vi "InitialiseProbeplan.vi"(8 "error in (no error)":errorcluster, 11 "ProbeStationControl in":refnum<class "ProbeStationControl.lvclass">) -> (0 "error out":errorcluster, 3 "ProbeStationControl out":refnum<class "ProbeStationControl.lvclass">)   [LabVIEW 2019]
doc: "General utility to initialise, generate, test and execute probe plans."
uses:
  InstrControl/ProbeStationControl/ProbeStationControl.lvclass
  ProbePlanParams.vi
  general_VIs/globals/QC_MeasurementSetup.vi
panel:
  in  "Continue":bool
  in  "New Sensor":bool
  in  "Single Needle":bool
  in  "Probe Card Channels":i32=32
  in  "Strip No.":u16(ring)
  out "Probeplan:":string
  in  "Region":u16(ring)
  in  "Chuck":bool caption="Chuck\nDOWN"
  in  "New Button":bool
  in  "Jump Button":bool
  out "Chuck Up/Down check":bool
  # "Probeplan"
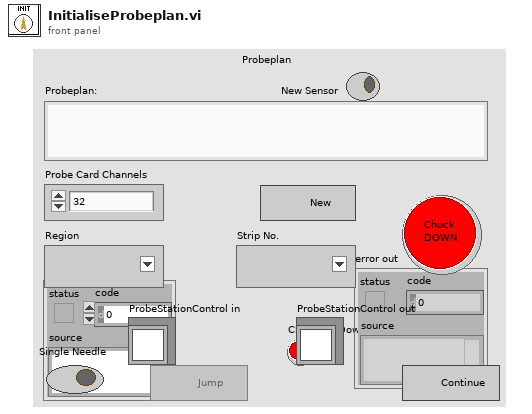
[diagram p1: front panel]
types:
  T1 = cluster{"Strip Number OUT":i32, "X0":i32, "Y0":i32, "X1":i32, "Y1":i32, "Xref":dbl, "Yref":dbl, "ProbePlan type":u32, "Inner pads offset":ext, "Outer pads offset":ext, "l_inner":ext, "l_outer":ext, "strip numbering":u16, "Device Orientation":ext, "Stagger offset":i32, "Yoffset":dbl, "Strip pitch":dbl, "Fiducail separation":dbl, "Radius":ext, "Relative strip angles":dbl, "Probeplan description":string, "ProbePlan array":cluster{"Region":string, "ProbePoints":cluster{"X":dbl, "Y":dbl, "Label":string, "CardViable?":bool}[]}[], "Test ProbePoints":cluster{"Regions Enabled":bool[], "From index":u32[], "To index":u32[]}}
  T2 = cluster{"Bias Supply":refnum<class "SupplyControl.lvclass">, "SMU":refnum<class "SupplyControl.lvclass">, "LCR":refnum<class "LCRControl.lvclass">, "Probe Card Channels":i32, "Bias Voltage [V]":dbl, "First strip":i32, "Last strip":i32, "Base Voltage [V]":dbl, "Base Ramp Step [V]":dbl, "Base Ramp Interval [ms]":u32, "High Voltage [V]":dbl, "High Ramp Step [V]":dbl, "High Ramp Interval [ms]":u32, "AC frequency [Hz]":i32, "AC amplitude [V]":dbl, "RC Configuration":u16, "Single Needle":bool, "Temperature Readout":enum16{"Read Arduino", "Enter manually"}, "Arduino":refnum<class "ArduinoControl.lvclass">, "Fraction of good strips [%]":dbl, "ProbeStation":refnum<class "ProbeStationControl.lvclass">, "Switching":refnum<class "Switching.lvclass">, "Matrix used?":bool, "Matrix X Channels":cluster{"Bias Supply / SMU LO":i32, "Bias Supply / SMU HI":i32, "CV Box LO":i32, "CV Box HI":i32, "CV Box LO IN":i32, "CV Box HI IN":i32, "Volt meter LO":i32, "Volt meter HI":i32, "Mux1 C1":i32, "Mux1 C2":i32, "Mux2 C1":i32, "Mux2 C2":i32}, "Pinholes Y/N":bool, "Capacitance Y/N":bool, "Resistance Y/N":bool, "Bias Supply Name":string, "SMU Name":string, "LCR Name":string}
  T3 = cluster{"Region":string, "ProbePoints":cluster{"X":dbl, "Y":dbl, "Label":string, "CardViable?":bool}[]}[]
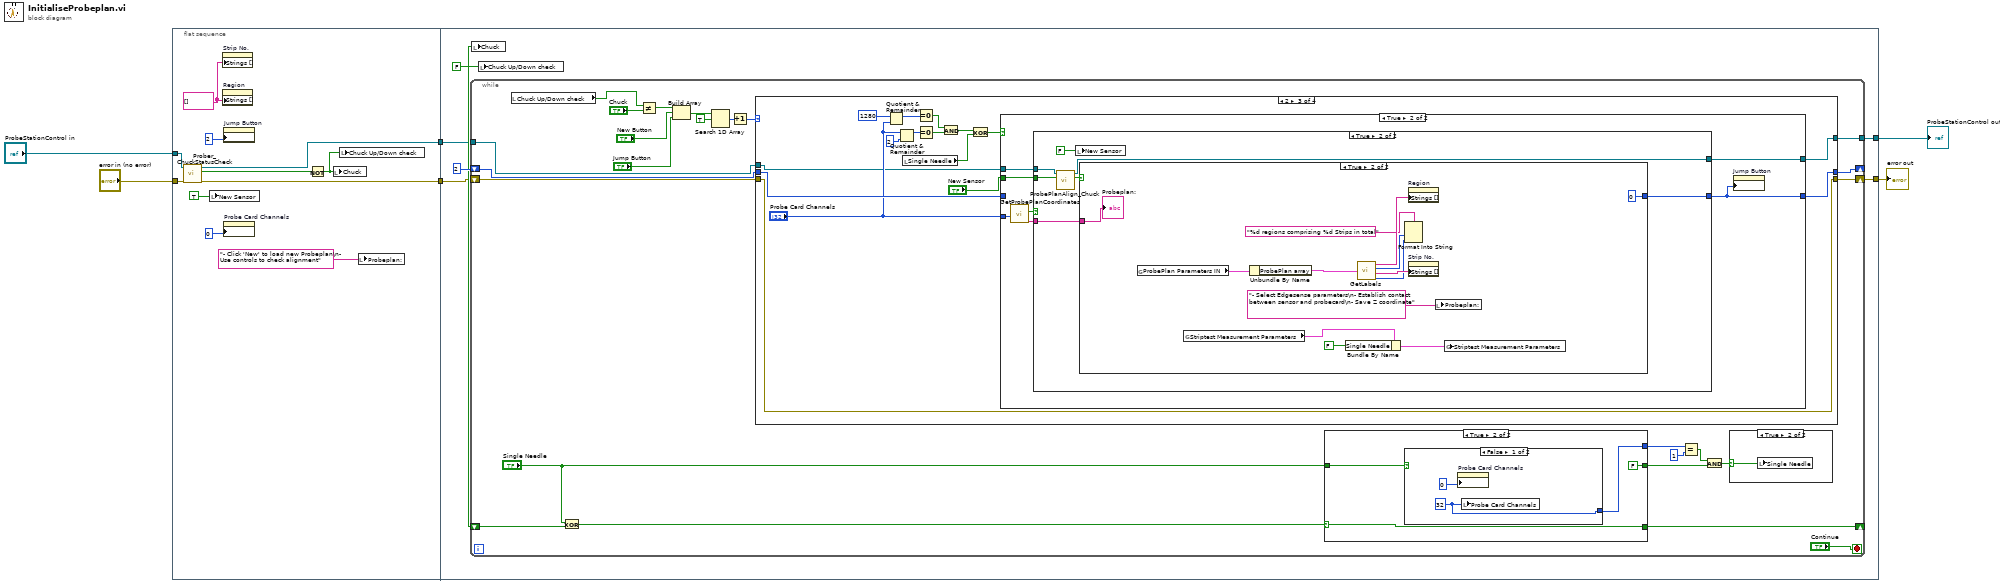
[diagram p0: block diagram]
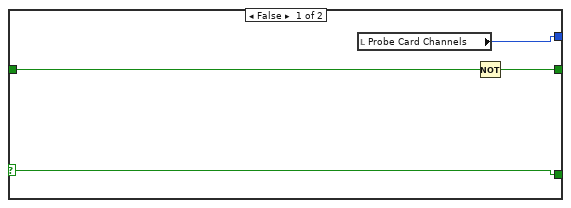
[diagram p3: hidden frame]
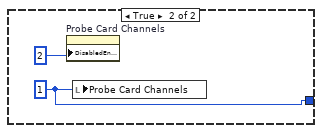
[diagram p4: hidden frame]
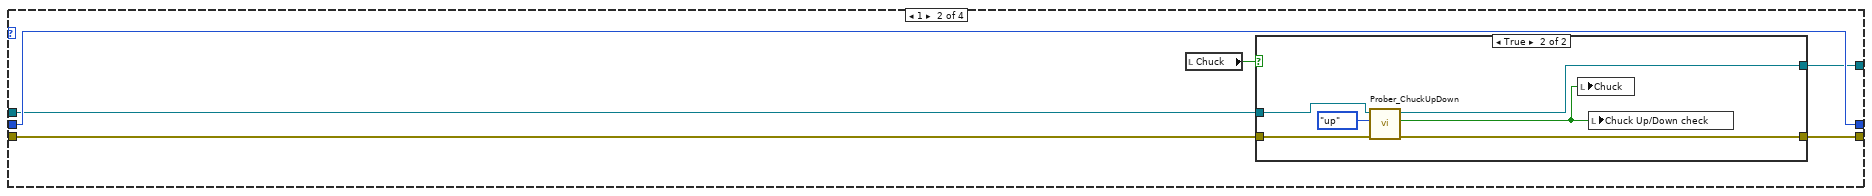
[diagram p6: hidden frame]
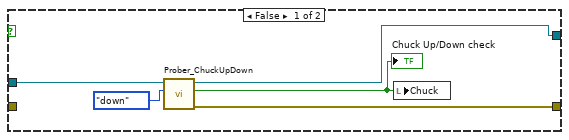
[diagram p7: hidden frame]
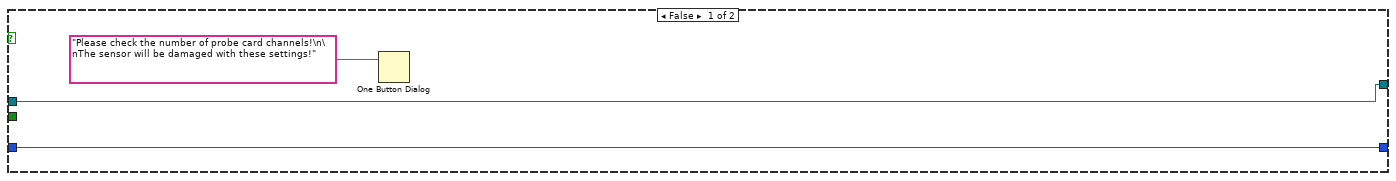
[diagram p8: hidden frame]
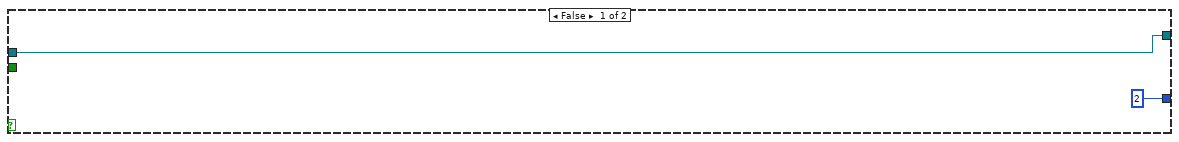
[diagram p9: hidden frame]
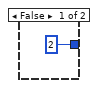
[diagram p10: hidden frame]
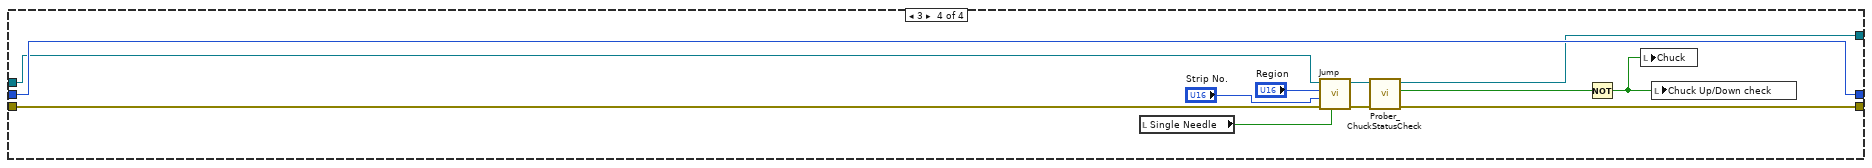
[diagram p11: hidden frame]
diagram:
  n1 = flat-sequence {
    tunnel: "ProbeStationControl in" -> [w11]
    tunnel: [w7] -> w3
    tunnel: "error in (no error)" -> [w9]
    tunnel: [w8] -> w2
    tunnel: w3 -> [w21]
    tunnel: [w20] -> w5
    tunnel: w2 -> [w19]
    tunnel: [w18] -> w1
    frame #0 {
      w15 = string[] []
      n2 = call-dynamic "Prober_ChuckStatusCheck.vi"("error in (no error)"=w9, "ProbeStationControl in"=w11) -> ("error out"=w8:errorcluster, "Chuck at CONTACT?"=w13:bool, "ProbeStationControl out"=w7:refnum<class "ProbeStationControl.lvclass">)  [unwired: 7 in]
      n3 = local write "New Sensor"(TRUE) -> ()
      n4 = property on="Strip No." class="Ring (strict)"("Strings []"=w15) -> ()  [unwired: 2 in, 2 out]
      n5 = property on="Region" class="Ring (strict)"("Strings []"=w15) -> ()  [unwired: 2 in, 2 out]
      n6 = property on="Jump Button" class="Bool"("DisabledEnum"=2) -> ()  [unwired: 2 in, 2 out]
      n7 = property on="Probe Card Channels" class="DigNum (strict)"("DisabledEnum"=0) -> ()  [unwired: 2 in, 2 out]
      n8 = Not(x=w13) -> (.not. x?=w12:bool)
      n9 = local write "Chuck"(w12) -> ()
      n10 = local write "Chuck Up/Down check"(w12) -> ()
      n11 = local write "Probeplan:"("- Click 'New' to load new Probeplan\n- Use controls to check alignment") -> ()
    }
    frame #1 {
      w22 = FALSE
      n12 = while {
        shift-right: [w41] -> _
        shift-left: 2 -> [w42]
        shift-right: [w29] -> _
        shift-left: w22 -> [w30]
        tunnel: w21 -> [w27]
        tunnel: [w26] -> w20
        shift-right: [w24] -> w18
        shift-left: w19 -> [w25]
        stop <- "Continue" stop-if-true
        n13 = local read "Chuck Up/Down check"() -> (w40:bool)
        n14 = Exclusive Or(1:w30, 2:"Single Needle") -> (0:w32:bool)
        n15 = Not Equal?(x=w40, y="Chuck") -> (x != y?=w38:bool)
        n16 = Build Array(w38, "New Button", "Jump Button") -> (w47:bool[])
        n17 = Search 1D Array(1D array=w47, element=TRUE) -> (index of element=w48:i32)  [unwired: 1 in]
        n18 = Increment(x=w48) -> (x+1=w43:i32)
        n19 = case shown="2" w43 {
          tunnel: w42 -> [w64 w70 w95 w142]
          tunnel: [w64 w70 w97 w142] -> w41
          tunnel: w27 -> [w63 w68 w87 w141]
          tunnel: [w63 w67 w86 w140] -> w26
          tunnel: w25 -> [w62 w65 w82 w136]
          tunnel: [w62 w66 w82 w138] -> w24
          frame 0, Default {
          }
          frame 1 {
            n20 = local read "Chuck"() -> (w69:bool)
            n21 = case shown="True" w69 {
              tunnel: w68 -> [w74 w79]
              tunnel: [w72 w78] -> w67
              tunnel: [w71 w77] -> w66
              tunnel: w65 -> [_ w76]
              frame False {
                n22 = call-dynamic "Prober_ChuckUpDown.vi"("Direction"=enum16{"up", "down"}."down", "ProbeStationControl in"=w74) -> ("error out"=w71:errorcluster, "Chuck at CONTACT?"=w75:bool, "ProbeStationControl out"=w72:refnum<class "ProbeStationControl.lvclass">)  [unwired: 7 in]
                "Chuck Up/Down check" <- w75
                n23 = local write "Chuck"(w75) -> ()
              }
              frame True {
                n24 = call-dynamic "Prober_ChuckUpDown.vi"("error in (no error)"=w76, "Direction"=enum16{"up", "down"}."up", "ProbeStationControl in"=w79) -> ("error out"=w77:errorcluster, "Chuck at CONTACT?"=w81:bool, "ProbeStationControl out"=w78:refnum<class "ProbeStationControl.lvclass">)  [unwired: 6 in]
                n25 = local write "Chuck"(w81) -> ()
                n26 = local write "Chuck Up/Down check"(w81) -> ()
              }
            }
          }
          frame 2 {
            n27 = Quotient & Remainder(x=1280, y="Probe Card Channels") -> (x-y*floor(x/y)=w96:i32)  [unwired: 1 out]
            n28 = Quotient & Remainder(x="Probe Card Channels", y=2) -> (x-y*floor(x/y)=w90:i32)  [unwired: 1 out]
            n29 = local read "Single Needle"() -> (w83:bool)
            n30 = Equal To 0?(x=w96) -> (x = 0?=w94:bool)
            n31 = Equal To 0?(x=w90) -> (x = 0?=w89:bool)
            n32 = And(x=w94, y=w89) -> (x .and. y?=w85:bool)
            n33 = Exclusive Or(1:w83, 2:w85) -> (0:w84:bool)
            n34 = case shown="True" w84 {
              tunnel: "Probe Card Channels" -> [_ w105]
              tunnel: [w98 w104] -> w97
              tunnel: w95 -> [w98 _]
              tunnel: "New Sensor" -> [_ w103]
              tunnel: w87 -> [w99 w102]
              tunnel: [w99 w101] -> w86
              frame False {
                n35 = One Button Dialog(message="Please check the number of probe card channels!\n\nThe sensor will be damaged with these settings!") -> ()  [unwired: 1 in, 1 out]
              }
              frame True {
                n36 = call "GetProbePlanCoordinates.vi"("Probe Card Channels"=w105) -> ("file path"=w106:string, "OK?"=w107:bool)  [unwired: 1 out]
                n37 = case shown="True" w107 {
                  tunnel: [2 w116] -> w104
                  tunnel: w106 -> [_ w114]
                  tunnel: w103 -> [_ w113]
                  tunnel: w102 -> [w108 w112]
                  tunnel: [w108 w111] -> w101
                  frame False {
                  }
                  frame True {
                    n38 = call "ProbePlanAlign_Chuck.vi"("New Sensor"=w113, "ProbeStationControl in"=w112) -> ("Accept/Quit"=w115:bool, "ProbeStationControl out"=w111:refnum<class "ProbeStationControl.lvclass">)  [unwired: 8 in]
                    n39 = local write "New Sensor"(FALSE) -> ()
                    n40 = case shown="True" w115 {
                      tunnel: [2 0] -> w116
                      tunnel: w114 -> [_ w129]
                      frame False {
                      }
                      frame True {
                        n41 = global read "ProbePlanParams.vi" "ProbePlan Parameters IN"() -> (w128:T1)
                        n42 = global read "QC_MeasurementSetup.vi" "Striptest Measurement Parameters"() -> (w119:T2)
                        n43 = Unbundle By Name(w128) -> ("ProbePlan array"=w127:T3)
                        n44 = Bundle By Name(cluster=w119, "Single Needle"=FALSE) -> (w118:T2)
                        n45 = call "GetLabels.vi"("Array"=w127) -> ("Region Labels"=w125:string[], "No. of regions"=w124:i32, "Strip Labels"=w126:string[], "No. of Points"=w123:i32)
                        n46 = Format Into String(format string="%d regions comprising %d Strips in total", w124, w123) -> ()  [unwired: 2 in, 2 out]
                        n47 = property on="Region" class="Ring (strict)"("Strings []"=w125) -> ()  [unwired: 2 in, 2 out]
                        n48 = property on="Strip No." class="Ring (strict)"("Strings []"=w126) -> ()  [unwired: 2 in, 2 out]
                        n49 = local write "Probeplan:"("- Select Edgesense parameters\n- Establish contact between sensor and probecard\n- Save Z coordinate") -> ()
                        n50 = global write "QC_MeasurementSetup.vi" "Striptest Measurement Parameters"(w118) -> ()
                        "Probeplan:" <- w129
                      }
                    }
                  }
                }
                n51 = property on="Jump Button" class="Bool"("DisabledEnum"=w104) -> ()  [unwired: 2 in, 2 out]
              }
            }
          }
          frame 3 {
            n52 = local read "Single Needle"() -> (w133:bool)
            n53 = call "Jump.vi"("Single Needle"=w133, "Error In"=w136, "Strip No."="Strip No.", "Region"="Region", "ProbeStationControl in"=w141) -> ("Error Out"=w137:errorcluster, "ProbeStationControl out"=w139:refnum<class "ProbeStationControl.lvclass">)  [unwired: 5 in]
            n54 = call-dynamic "Prober_ChuckStatusCheck.vi"("error in (no error)"=w137, "ProbeStationControl in"=w139) -> ("error out"=w138:errorcluster, "Chuck at CONTACT?"=w132:bool, "ProbeStationControl out"=w140:refnum<class "ProbeStationControl.lvclass">)  [unwired: 7 in]
            n55 = Not(x=w132) -> (.not. x?=w131:bool)
            n56 = local write "Chuck"(w131) -> ()
            n57 = local write "Chuck Up/Down check"(w131) -> ()
          }
        }
        n58 = case shown="True" w32 {
          selector: w32 -> [w50 w54]
          tunnel: [w52 FALSE] -> w35
          tunnel: [w53 w56] -> w33
          tunnel: "Single Needle" -> [w51 w55]
          tunnel: [w50 w54] -> w29
          frame False {
            n59 = local read "Probe Card Channels"() -> (w53:i32)
            n60 = Not(x=w51) -> (.not. x?=w52:bool)
          }
          frame True {
            n61 = case shown="False" w55 {
              tunnel: [w58 w61] -> w56
              frame False {
                w58 = 32
                n62 = property on="Probe Card Channels" class="DigNum (strict)"("DisabledEnum"=0) -> ()  [unwired: 2 in, 2 out]
                n63 = local write "Probe Card Channels"(w58) -> ()
              }
              frame True {
                w61 = 1
                n64 = property on="Probe Card Channels" class="DigNum (strict)"("DisabledEnum"=2) -> ()  [unwired: 2 in, 2 out]
                n65 = local write "Probe Card Channels"(w61) -> ()
              }
            }
          }
        }
        n66 = Equal?(x=w33, y=1) -> (x = y?=w36:bool)
        n67 = And(x=w36, y=w35) -> (x .and. y?=w34:bool)
        n68 = case shown="True" w34 {
          selector: w34 -> [_ w49]
          frame False {
          }
          frame True {
            n69 = local write "Single Needle"(w49) -> ()
          }
        }
      }
      n70 = local write "Chuck"(w22) -> ()
      n71 = local write "Chuck Up/Down check"(w22) -> ()
    }
  }
  "ProbeStationControl out" <- w5
  "error out" <- w1
